vi "json Close.vi"(8 "error in (no error)":errorcluster, 11 "JSON Document in":refnum<class "JSON Document.lvclass">) -> (0 "error out":errorcluster)   [LabVIEW 2015, in "JSON Document.lvclass"]
uses:
  JSON Document.lvclass
  JSON Document.lvclass/JSON Document.ctl
  rapidjson wrapper/rapidjson wrapper.lvlib
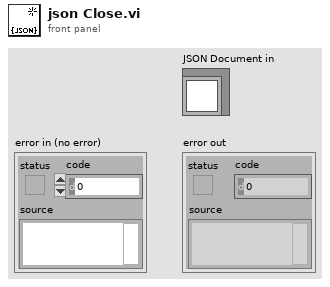
[diagram p1: front panel]
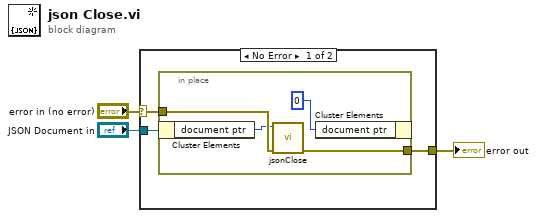
[diagram p0: block diagram]
diagram:
  n1 = case shown="No Error" "error in (no error)" {
    selector: "error in (no error)" -> [w6 w11]
    tunnel: [w5 w11] -> w2
    tunnel: "JSON Document in" -> [w4 _]
    frame No Error {
      n2 = in-place {
        in-place-border: w6 -> [w10]
        in-place-border: [w9] -> w5
        n3 = in-place-cluster #1(w4) -> ("document ptr"=w8:i64)
        n4 = call "jsonClose.vi"("error in (no error)"=w10, "d"=w8) -> ("error out"=w9:errorcluster)  [unwired: 9 in]
        n5 = in-place-cluster #1("document ptr"=i64 0) -> ()  [unwired: 1 out]
      }
    }
    frame Error {
    }
  }
  "error out" <- w2
